vi "GetAttributeViInt32_Advanced.vi"(8 "error in (no error)":errorcluster {"code" format="%.0x"}, 9 "AttributeID":u32(ring)=1950001 items=["IVILXISYNC_ARM_ALARM_COUNT"=1950001, "IVILXISYNC_ARM_ALARM_REPEAT_COUNT"=1950004, "IVILXISYNC_ARM_COUNT"=1950007, "IVILXISYNC_ARM_SOURCE_COUNT"=1950009, "IVILXISYNC_ARM_SOURCE_DETECTION"=1950010, "IVILXISYNC_EVENT_COUNT"=1950028, "IVILXISYNC_EVENT_DRIVE_MODE"=1950030, "IVILXISYNC_EVENT_LOG_ENTRY_COUNT"=1950035, "IVILXISYNC_EVENT_SLOPE"=1950031, "IVILXISYNC_EVENT_WIRED_OR_BIAS_MODE"=1950033, "IVILXISYNC_TRIGGER_ALARM_COUNT"=1950015, "IVILXISYNC_TRIGGER_ALARM_REPEAT_COUNT"=1950018, "IVILXISYNC_TRIGGER_COUNT"=1950021, "IVILXISYNC_TRIGGER_SOURCE_COUNT"=1950023, "IVILXISYNC_TRIGGER_SOURCE_DETECTION"=1950025, "LEVEL_ATTENUATION_OPTIMIZE"=1150012, "LEVEL_ATTENUATION_STEP_INCREMENT"=1150013, "LEVEL_ELECTRONIC_ATTENUATION"=1150578, "MARKER_COUNT"=1250203, "MARKER_TYPE"=1250701, "MEMORYOPERATION_SCREEN_IMAGE_THEME"=1150678, "NUMBER_OF_DIVISIONS"=1250602, "NUMBER_OF_SWEEPS"=1250010, "OUTPUT_ANALOG_TYPE"=1150679, "OUTPUT_AUXILIARY_IF_TYPE"=1150681, "PRESELECTOR_MW_PATH"=1150585, "RADIO_BAND_CLASS"=1150550, "RADIO_DEVICE"=1150547, "RADIO_NON_STANDARD_MEASUREMENT_ENABLED"=1150549, "RADIO_PACKET_TYPE"=1150551, "RADIO_STANDARD"=1150548, "REFOSCILLATOR_EXTERNAL_BANDWIDTH"=1150539, "REFOSCILLATOR_EXTERNAL_COUPLING"=1150538, "REFOSCILLATOR_SOURCE"=1150877, "STATETRIGGER_DETECTION"=1150159, "STATUS_SERIAL_POLL"=1150759, "SYSTEM_IO_TIMEOUT"=1150783, "SYSTEM_TIMEOUT_MILLISECONDS"=1150175, "TRACE_COUNT"=1250018, "TRACE_DETECTOR_TYPE"=1150782, "TRACE_SIZE"=1250019, "TRACE_TYPE"=1250020, "TRACES_AVERAGE_TYPE"=1150666, "TRIGGER_EXTERNAL2_SLOPE"=1150671, "TRIGGER_EXTERNAL_SLOPE"=1150803, "TRIGGER_FRAME_SYNC_SOURCE "=1150841, "TRIGGER_LINE_DELAY_SLOPE "=1150836, "TRIGGER_RFBURST_SLOPE"=1150830, "TRIGGER_SOURCE"=1250301, "TRIGGER_VIDEO_SLOPE"=1150806, "VERTICAL_SCALE"=1250021, "VIDEO_TRIGGER_SLOPE"=1250502], 10 "RepCapIdentifier":string, 11 "instrument handle":refnum<k15>) -> (0 "error out":errorcluster {"code" format="%.0x"}, 2 "AttributeValue":i32, 3 "instrument handle out":refnum<k15>)   [LabVIEW 2009, in "Keysight XSAn.lvlib"]
doc: "Gets an Int32 attribute from the instrument driver.\nThe following Attributes are supported:\n\nIVILXISYNC_ARM_ALARM_COUNT\nIVILXISYNC_ARM_ALARM_REPEAT_COUNT\nIVILXISYNC_ARM_COUNT\nIVILXISYNC_ARM_SOURCE_COUNT\nIVILXISYNC_ARM_SOURCE_DETECTION\nIVILXISYNC_EVENT_COUNT\nIVILXISYNC_EVENT_DRIVE_MODE\nIVILXISYNC_EVENT_LOG_ENTRY_COUNT\nIVILXISYNC_EVENT_SLOPE\nIVILXISYNC_EVENT_WIRED_OR_BIAS_MODE\nIVILXISYNC_TRIGGER_ALARM_COUNT\nIVILXISYNC_TRIGGER_ALARM_REPEAT_COUNT\nIVILXISYNC_TRIGGER_COUNT\nIVILXISYNC_TRIGGER_SOURCE_COUNT\nIVILXISYNC_TRIGGER_SOURCE_DETECTION\nLEVEL_ATTENUATION_OPTIMIZE\nLEVEL_ATTENUATION_STEP_INCREMENT\nLEVEL_ELECTRONIC_ATTENUATION\nMARKER_COUNT\nMARKER_TYPE\nMEMORYOPERATION_SCREEN_IMAGE_THEME\nNUMBER_OF_DIVISIONS\nNUMBER_OF_SWEEPS\nOUTPUT_ANALOG_TYPE\nOUTPUT_AUXILIARY_IF_TYPE\nPRESELECTOR_MW_PATH\nRADIO_BAND_CLASS\nRADIO_DEVICE\nRADIO_NON_STANDARD_MEASUREMENT_ENABLED\nRADIO_PACKET_TYPE\nRADIO_STANDARD\nREFOSCILLATOR_EXTERNAL_BANDWIDTH\nREFOSCILLATOR_EXTERNAL_COUPLING\nREFOSCILLATOR_SOURCE \nSTATETRIGGER_DETECTION\nSTATUS_SERIAL_POLL\nSYSTEM_IO_TIMEOUT\nSYSTEM_TIMEOUT_MILLISECONDS\nTRACE_COUNT\nTRACE_DETECTOR_TYPE\nTRACE_SIZE\nTRACE_TYPE\nTRACES_AVERAGE_TYPE\nTRIGGER_EXTERNAL2_SLOPE\nTRIGGER_EXTERNAL_SLOPE\nTRIGGER_FRAME_SYNC_SOURCE\nTRIGGER_LINE_DELAY_SLOPE\nTRIGGER_RFBURST_SLOPE\nTRIGGER_SOURCE\nTRIGGER_VIDEO_SLOPE\nVERTICAL_SCALE\nVIDEO_TRIGGER_SLOPE"
uses:
  <instrlib>/Keysight XSAn/Keysight XSAn.lvlib
  AgXSAn.dll
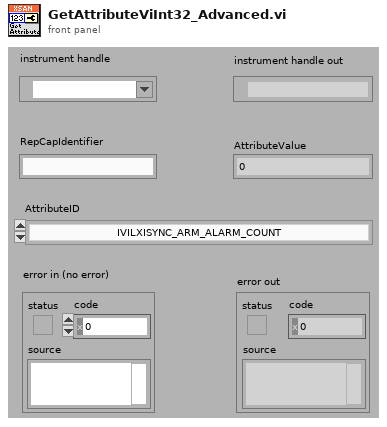
[diagram p1: front panel]
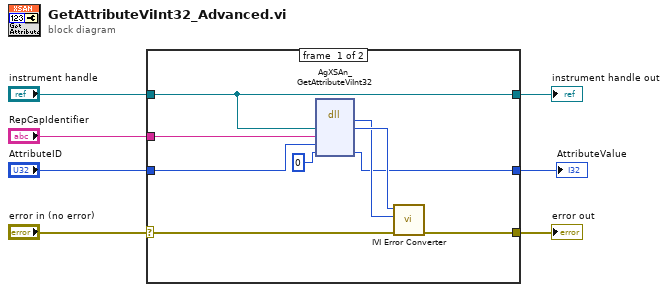
[diagram p0: block diagram]
diagram:
  n1 = case shown="No Error" "error in (no error)" {
    selector: "error in (no error)" -> [w14 w18]
    tunnel: [w13 w18] -> w7
    tunnel: "instrument handle" -> [w8 w17]
    tunnel: "RepCapIdentifier" -> [w12 _]
    tunnel: "AttributeID" -> [w11 _]
    tunnel: [w9 _] -> w2
    tunnel: [w8 w17] -> w1
    frame #0 {
      n2 = dll-call lib="AgXSAn**.dll" fn="AgXSAn_GetAttributeViInt32"("Vi"=w8, "RepCapIdentifier"=w12, "AttributeID"=w11, "AttributeValue"=0) -> ("return type"=w15:i32, "Vi"=w16:u32, "AttributeValue"=w9:i32)  [unwired: 5 in, 2 out]
      n3 = call <instrlib>:"IVI Error Converter.vi"("error in (no error)"=w14, "IVI error code (0)"=w15, "instrument handle"=w16) -> ("error out"=w13:errorcluster)  [unwired: 7 in, 1 out]
    }
    frame #1 {
    }
  }
  "error out" <- w7
  "instrument handle out" <- w1
  "AttributeValue" <- w2
